vi "APC_9049_FPGA_main.vi"() -> ()   [LabVIEW 2020]
uses:
  <vilib>/Platform/TimedLoop/XDataNode/timing_clust.ctl
  <vilib>/Platform/TimedLoop/XDataNode/nitl_modes.ctl
  <vilib>/Platform/TimedLoop/XDataNode/wakeup.ctl
  <vilib>/rvi/eio/common/nirviEmuTemplateMethod_errors.vi
  <vilib>/rvi/Emulation/niFpgaGetClockAttributes.vi
  <vilib>/rvi/Emulation/niFpgaSctlEmulationGetInTimedLoop.vi
  <vilib>/rvi/Emulation/niFpgaEmulationReportErrorSimple.vi
  <vilib>/rvi/Emulation/niFpgaCriticalErrorInLSC.vi
  <vilib>/Powertrain Controls/Device Drivers/Engine Position Tracking/RevC/Encoder/FPGA/ept_enc_vte2_revc.vi
  <vilib>/eio/EIOMethodNode/EIOMethodNode.xnode
  <vilib>/eio/EIONode/EIONode.xnode
  <vilib>/Platform/TimedLoop/XDataNode/XDataNode.xnode
  <vilib>/Platform/TimedLoop/XDataNode/XDNodeRunTimeDep.lvlib
panel:
  out "Finished Late? [i-1]":bool
  out "CrankCount":u16
  out "NumberOfActiveIGN_DI":u8
  in  "manual toggle mode?":bool
  in  "Time out limit":u32=6000000
  in  "manual?":bool
  in  "PFI0 manual OUT":bool
  in  "broadcast inj+ign?":bool
  out "PFI0 DO":bool
  in  "Ticks per toggle":u32[](array[numeric])=[13000, 12000, 11000, 10000, 9000, 8000, 7000, 6000, 5000, 4000, 3000, 2000, 1000]
  in  "Toggle mode":u8
  in  "toggle TDC":bool
  in  "1/2 Z pulse":bool
  in  "Mod3/DIO7":bool
  in  "Mod3/DIO6":bool
  in  "Mod3/DIO5":bool
  in  "Mod3/DIO4":bool
  in  "Mod4/DIO7":bool
  in  "Mod4/DIO6":bool
  in  "DI 4":T1
  in  "DI 5":T1
  in  "DI 6":T1
  out "DI_Data_Mod6":T2 caption="DIData"
  in  "DI 1":T1
  in  "DI 2":T1
  in  "DI 3":T1
  in  "Spark 6":T3
  in  "Spark 5":T3
  in  "Spark 4":T3
  in  "Spark 3":T3
  in  "Spark 2":T3
  out "Cam_sim":bool
  out "EncZ_w_offset":bool
  in  "TRIG1_offset_ticks":u16=2
  in  "Cam_tooth_w_ticks":u16=8
  in  "filt_crank A_ticks":u16=2
  in  "Must Use Cam & Z":bool
  out "CamZ filt":bool
  in  "filt_cam_ticks":u16
  out "Cam":bool
  out "EncZ":bool=TRUE
  out "EncB":bool=TRUE
  out "EncA":bool
  in  "filt_crank Z_ticks":u16
  out "dT HB (ms)":u32=500
  out "dT inj (ticks)":u32=1
  out "FPGA Heartbeat":bool=TRUE
  out "Chassis Temp Raw (x4 C)":i16=140
  out "SparkOut":bool
  in  "Spark 1":T3
  in  "DI_IPhaseInterface":T4(array[cluster]) caption="IPhaseInterface"
  in  "DI_Control":T5={"ModuleEnable"=FALSE, "WatchdogIn"=TRUE, "OneShotSelect"=enum."DISABLED", "OneShotTime"=40000, "OneShot"=FALSE, "Control"=0, "Control2"=128, "HostMode"=0, "HostCommand"=0, "HVTarget"=124, "BackBoostTime"=10, "Fault_ClrSig"=FALSE} caption="DIControl"
  out "DI_Data_Mod5":T2 caption="DIData"
  out "NI9401 Ready":bool=TRUE
  out "EPTOutSig":cluster{"CrankSigOut":bool, "CamSigOut":bool}
  out "EPTData":T6={"CrankSigOS"=FALSE, "CrankStalled"=FALSE, "SyncStopped"=FALSE, "MissedCrankFlag"=FALSE, "MissedCamFlag"=FALSE, "Period"=588, "PeriodAccum"=3882066, "CrankCount"=5844, "CurrentPosition"=23376, "MAX_CAT"=57600}
  in  "EPTControl":T7={"NumberOfCrankTeeth"=7200, "Stroke (FALSE=2, TRUE=4)"=TRUE, "CrankStallPeriod"=5000000, "CrankCountStart"=7200, "PeriodAccumCount"=7200, "SyncEnable"=TRUE, "SimEnable"=FALSE, "MissedCrankFlagClr"=TRUE, "MissedCamFlagClr"=TRUE, "SimPeriod"=500, "WatchdogIn"=TRUE}
  # "This is low level FPGA interface only! - DO NOT USE DIRECTLY - Use RT module to configure"
  # "DI Control"
  # "ENCODER SIGNAL"
  # "DI Driver Settings"
  # "monarch APC v0.1"
  # "cRIO 9049 FPGA"
  # "General Monitoring & Control"
  # "USER LED1 is also \nbroadcasting the \nhearbeat at 1Hz"
  # "Additional DO"
  # "Ignition Control"
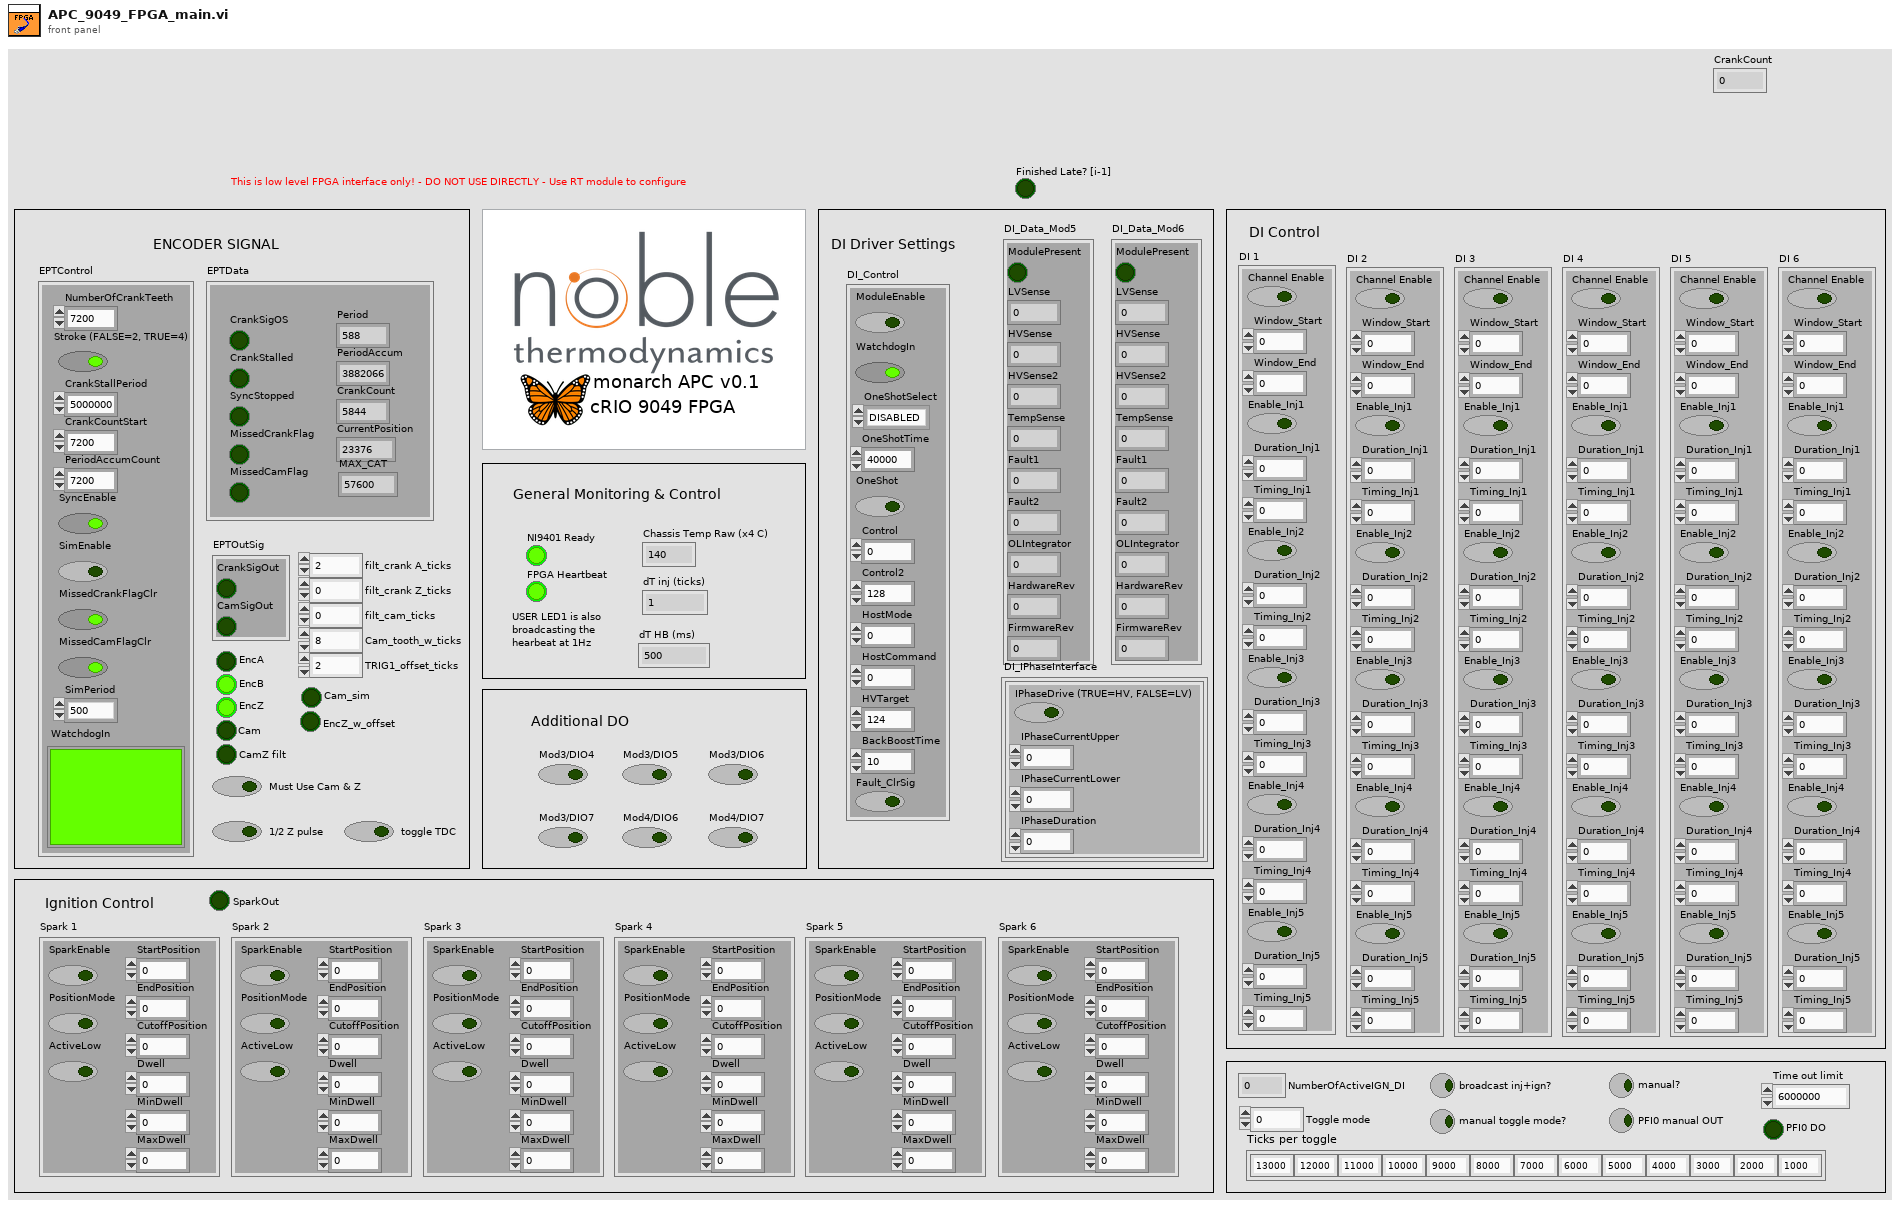
[diagram p1: front panel]
types:
  T1 = cluster{"Channel Enable":bool, "Window_Start":u16, "Window_End":u16, "Enable_Inj1":bool, "Duration_Inj1":u32, "Timing_Inj1":u16, "Enable_Inj2":bool, "Duration_Inj2":u32, "Timing_Inj2":u16, "Enable_Inj3":bool, "Duration_Inj3":u32, "Timing_Inj3":u16, "Enable_Inj4":bool, "Duration_Inj4":u32, "Timing_Inj4":u16, "Enable_Inj5":bool, "Duration_Inj5":u32, "Timing_Inj5":u16}
  T2 = cluster{"ModulePresent":bool, "LVSense":u8, "HVSense":u8, "HVSense2":u8, "TempSense":i8, "Fault1":u8, "Fault2":u8, "OLIntegrator":u32, "HardwareRev":u8, "FirmwareRev":u8}
  T3 = cluster{"SparkEnable":bool, "PositionMode":bool, "ActiveLow":bool, "StartPosition":u16, "EndPosition":u16, "CutoffPosition":u16, "Dwell":u32, "MinDwell":u32, "MaxDwell":u32}
  T4 = cluster{"IPhaseDrive (TRUE=HV, FALSE=LV)":bool, "IPhaseCurrentUpper":u16, "IPhaseCurrentLower":u16, "IPhaseDuration":u16}[]
  T5 = cluster{"ModuleEnable":bool, "WatchdogIn":bool, "OneShotSelect":enum8{"DISABLED", "CHAN 1", "CHAN 2", "CHAN 3"}, "OneShotTime":u32, "OneShot":bool, "Control":u8, "Control2":u8, "HostMode":u8, "HostCommand":u32, "HVTarget":u8, "BackBoostTime":u8, "Fault_ClrSig":bool}
  T6 = cluster{"CrankSigOS":bool, "CrankStalled":bool, "SyncStopped":bool, "MissedCrankFlag":bool, "MissedCamFlag":bool, "Period":u32, "PeriodAccum":u32, "CrankCount":u16, "CurrentPosition":u16, "MAX_CAT":u16}
  T7 = cluster{"NumberOfCrankTeeth":u16, "Stroke (FALSE=2, TRUE=4)":bool, "CrankStallPeriod":u32, "CrankCountStart":u16, "PeriodAccumCount":u16, "SyncEnable":bool, "SimEnable":bool, "MissedCrankFlagClr":bool, "MissedCamFlagClr":bool, "SimPeriod":u32, "WatchdogIn":bool}
  T8 = typedef "XDNodeRunTimeDep.lvlib/timing_clust.ctl" = cluster{"Expected End [f-1]":u64, "Actual End [f-1]":u64, "Finished Late? [f-1]":bool, "Expected End [i-1]":u64, "Actual End [i-1]":u64, "Finished Late? [i-1]":bool, "Expected Start [i]":u64, "Actual Start [i]":u64, "Expected Start [f]":u64, "Actual Start [f]":u64, "Source Name":string, "Structure Name":string, "Period":i64, "Deadline":i64, "Offset":i64, "Start":i64, "Priority":i32, "Timeout":i32, "Mode":T9, "Wakeup Reason":T10, "Error":errorcluster, "Source Type":string, "Secondary Source Type":string, "Global End Time":u64, "Global Start Time":u64, "Frame Duration":u64, "Iteration Duration":u64, "Assigned CPU":i32, "I/O Scan Engine Mode":u32}
  T9 = typedef "XDNodeRunTimeDep.lvlib/nitl_modes.ctl" = enum32{"No Change", "Process missed periods, maintain original phase", "Discard missed periods, maintain original phase", "Process missed periods, ignore original phase", "Discard missed periods, ignore original phase"}
  T10 = typedef "XDNodeRunTimeDep.lvlib/wakeup.ctl" = enum32{"Normal", "Aborted", "Asynchronous wakeup", "Timing source error", "Timed loop error", "Timeout"}
  T11 = cluster{"FSSup0":bool, "FSSup1":bool, "FSSup2":bool, "FSSup3":u16, "FSSup4":u32, "FSSup5":u16}
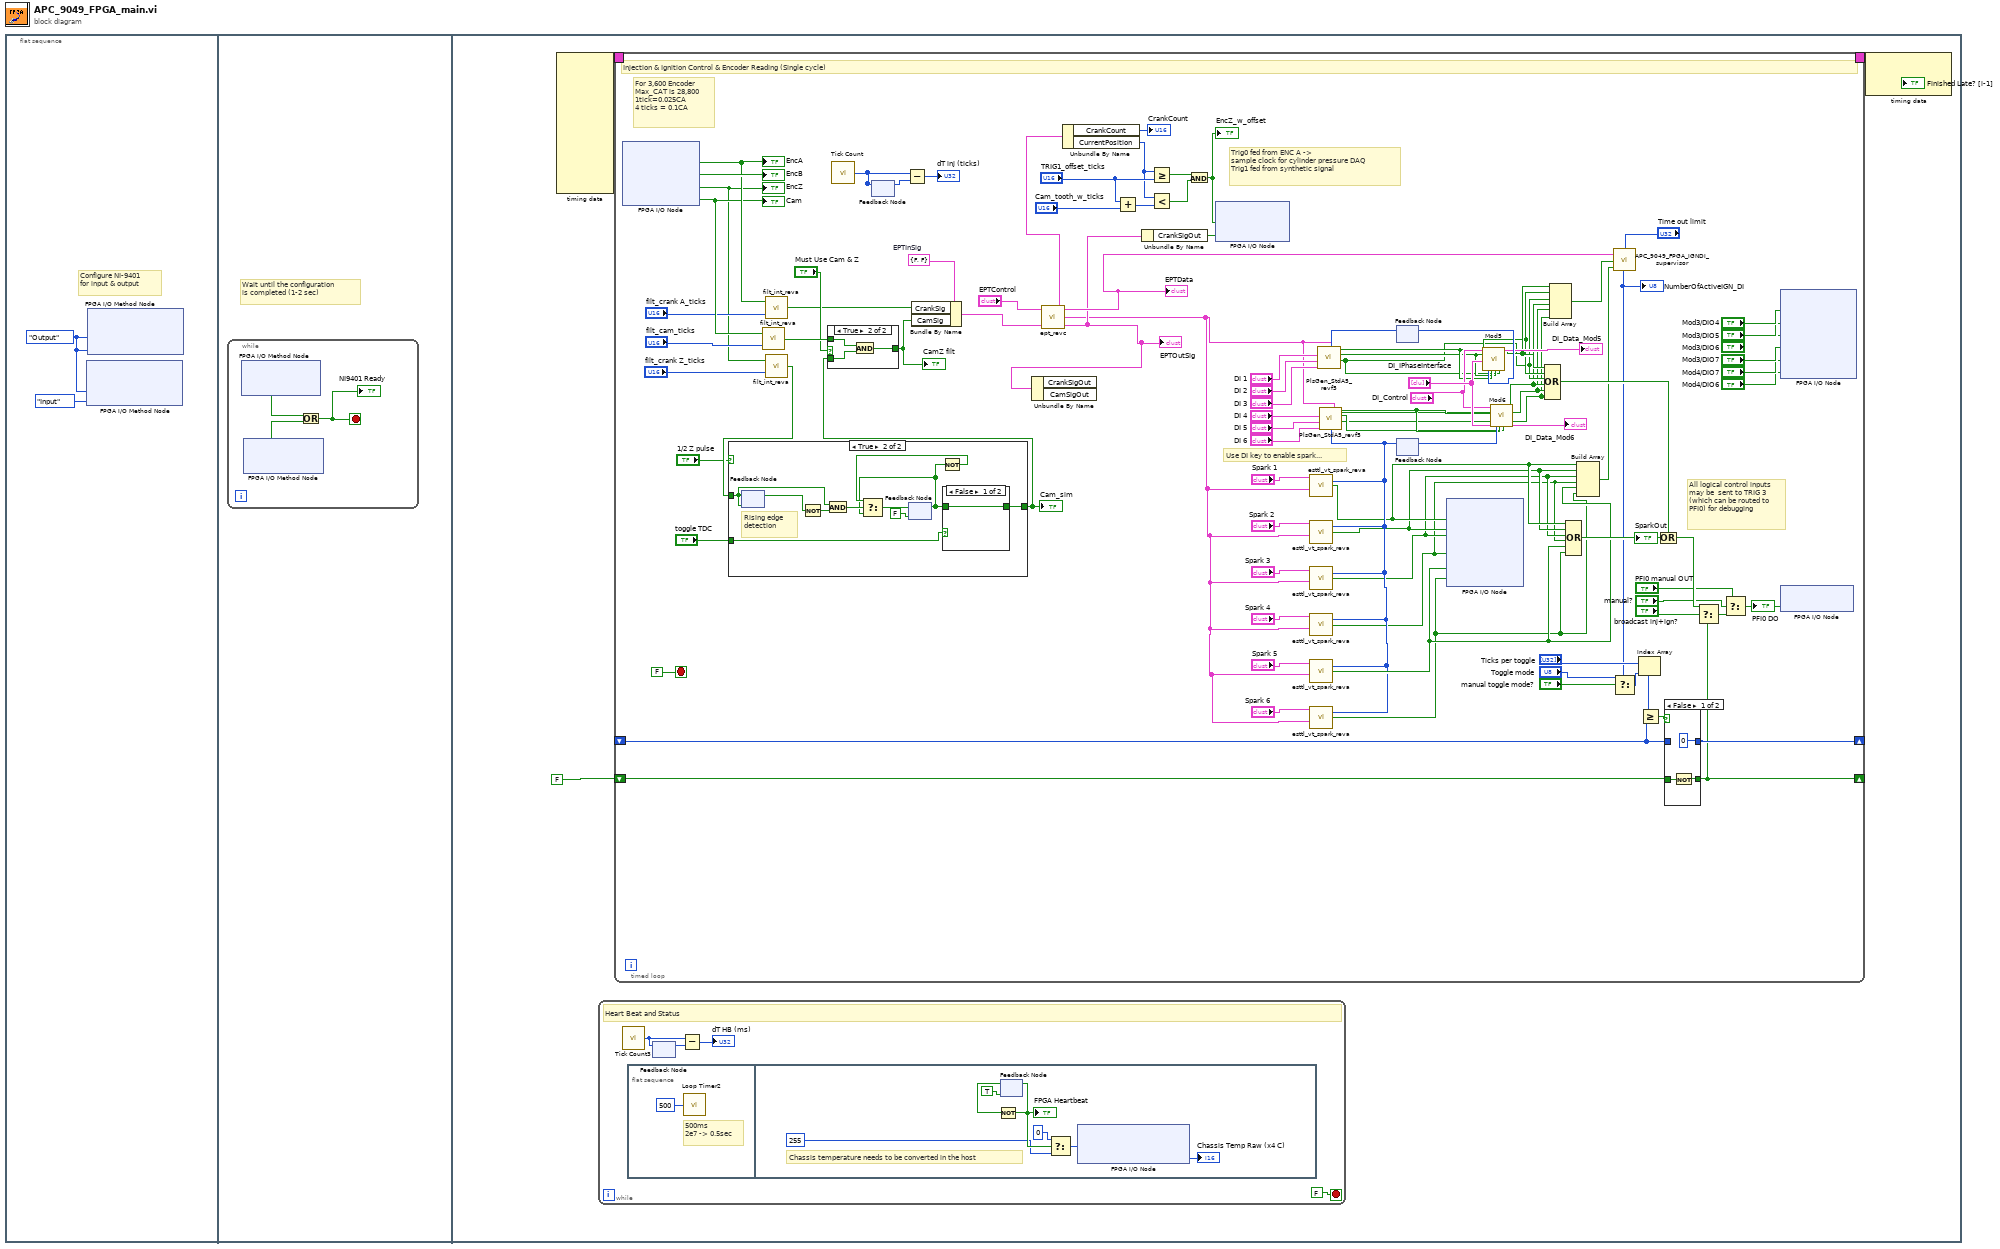
[diagram p0: block diagram]
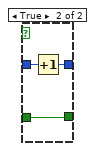
[diagram p2: hidden frame]
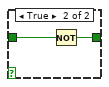
[diagram p4: hidden frame]
diagram:
  n1 = flat-sequence {
    frame #0 {
      w1 = enum8{"No Change", "Input", "Output"}."Output" ("DIO 7:4")
      # "Configure NI-9401 \nfor input & output"
      n2 = xnode "FPGA I/O Method Node"("DIO 7:4"=w1, "DIO 3:0"=enum8{"No Change", "Input", "Output"}."Input" ("DIO 7:4")) -> ()  [unwired: 1 in, 1 out]
      n3 = xnode "FPGA I/O Method Node"("DIO 7:4"=w1, "DIO 3:0"=w1) -> ()  [unwired: 1 in, 1 out]
    }
    frame #1 {
      # "Wait until the configuration \nis completed (1-2 sec)"
      n4 = while {
        stop <- w3 stop-if-true
        n5 = xnode "FPGA I/O Method Node"() -> ("Ready"=w5:bool)  [unwired: 1 in, 1 out]
        n6 = xnode "FPGA I/O Method Node"() -> ("Ready"=w4:bool)  [unwired: 1 in, 1 out]
        n7 = Or(x=w5, y=w4) -> (x .or. y?=w3:bool)
        "NI9401 Ready" <- w3
      }
    }
    frame #2 {
      n8 = node-c288() -> (w9:T8)  [unwired: 10 in]
      n9 = while {
        stop <- FALSE stop-if-true
        # "Heart Beat and Status"
        n10 = call "Tick Count3"() -> ("Tick Count(mSec)"=w12:u16)
        n11 = flat-sequence {
          frame #0 {
            # "500ms\n2e7 -> 0.5sec"
            n12 = call "Loop Timer2"("Count(mSec)"=u32 500) -> ()  [unwired: 1 out]
          }
          frame #1 {
            # "Chassis temperature needs to be converted in the host"
            n13 = feedback #1(TRUE ("USER FPGA LED")) -> (w19:bool)
            n14 = Not(x=w19) -> (.not. x?=w18:bool)
            "FPGA Heartbeat" <- w18
            n15 = feedback-in #1(w18) -> ()
            n16 = Select(t=u8 0, s=w18, f=u8 255) -> (s? t:f=w17:u8)
            n17 = xnode "FPGA I/O Node"("USER FPGA LED"=w17) -> ("Chassis Temperature"=→"Chassis Temp Raw (x4 C)":i16)  [unwired: 2 in, 2 out]
          }
        }
        n18 = feedback #2() -> (w13:u16)  [unwired: 1 in]
        n19 = feedback-in #2(w12) -> ()
        n20 = Subtract(x=w12, y=w13) -> (x-y=→"dT HB (ms)":u16)
      }
      n21 = timed-loop {
        timing-out: [_] -> w8
        timing: w9 -> [_]
        shift-right: [w73] -> _
        shift-left: _ -> [w72]
        shift-right: [w45] -> _
        shift-left: FALSE ("PFI0 mode signal") -> [w71]
        stop <- FALSE stop-if-true
        w109 = cluster{"CrankSig":bool, "CamSig":bool} {"CrankSig"=FALSE, "CamSig"=FALSE}  # EPTInSig
        # "All logical control inputs may be  sent to TRIG 3 (which can be routed to PFI0) for debugging"
        # "For 3,600 Encoder\nMax_CAT is 28,800\n1tick=0.025CA\n4 ticks = 0.1CA"
        # "Trig0 fed from ENC A -> \nsample clock for cylinder pressure DAQ\nTrig1 fed from synthetic signal"
        # "Use DI key to enable spark..."
        # "Injection & Ignition Control & Encoder Reading (Single cycle)"
        n22 = xnode "FPGA I/O Node"() -> ("Mod3/DIO0"=w107:bool, "Mod3/DIO1"=→"EncB":bool, "Mod3/DIO2"=w92:bool, "Mod3/DIO3"=w106:bool)  [unwired: 4 in, 4 out]
        "EncA" <- w107
        "EncZ" <- w92
        "Cam" <- w106
        n23 = call <vilib>:"filt_int_reva.vi"("FiltValue"="filt_cam_ticks", "InpSig"=w106) -> ("OutSig"=w103:bool)
        n24 = call <vilib>:"filt_int_reva.vi"("FiltValue"="filt_crank A_ticks", "InpSig"=w107) -> ("OutSig"=w38:bool)
        n25 = call <vilib>:"filt_int_reva.vi"("FiltValue"="filt_crank Z_ticks", "InpSig"=w92) -> ("OutSig"=w91:bool)
        n26 = case shown="True" "1/2 Z pulse" {
          tunnel: w91 -> [w122 w127]
          tunnel: [w122 w123] -> w40
          tunnel: "toggle TDC" -> [_ w125]
          frame False {
          }
          frame True {
            # "Rising edge \ndetection"
            n27 = feedback #3(w127) -> (w132:bool)
            n28 = feedback-in #3(w127) -> ()
            n29 = Not(x=w132) -> (.not. x?=w131:bool)
            n30 = And(x=w127, y=w131) -> (x .and. y?=w126:bool)
            n31 = feedback #4(FALSE) -> (w124:bool)
            n32 = Not(x=w124) -> (.not. x?=w130:bool)
            n33 = Select(t=w130, s=w126, f=w124) -> (s? t:f=w129:bool)
            n34 = feedback-in #4(w129) -> ()
            n35 = case shown="False" w125 {
              tunnel: w124 -> [w133 w135]
              tunnel: [w133 w134] -> w123
              frame False {
              }
              frame True {
                n36 = Not(x=w135) -> (.not. x?=w134:bool)
              }
            }
          }
        }
        "Cam_sim" <- w40
        n37 = case shown="True" "Must Use Cam & Z" {
          tunnel: w103 -> [_ w139]
          tunnel: w40 -> [w136 w138]
          tunnel: [w136 w137] -> w39
          frame False {
          }
          frame True {
            n38 = And(x=w139, y=w138) -> (x .and. y?=w137:bool)
          }
        }
        "CamZ filt" <- w39
        n39 = call "Tick Count"() -> ("Tick Count(Ticks)"=w112:u32)
        n40 = feedback-in #5(w112) -> ()
        n41 = feedback #5(w112) -> (w113:u32)
        n42 = Subtract(x=w112, y=w113) -> (x-y=→"dT inj (ticks)":u32)
        n43 = Bundle By Name(cluster=w109, "CrankSig"=w38, "CamSig"=w39) -> (w108:cluster{"CrankSig":bool, "CamSig":bool})
        n44 = call-poly <vilib>:"ept_revc.vi"("EPTControl"="EPTControl", "EPTInSig"=w108) -> ("EPTData"=w47:T6, "FuelSparkSupervisor"=w22:T11, "EPTOutSig"=w37:cluster{"CrankSigOut":bool, "CamSigOut":bool})  [unwired: 3 in]
        "EPTData" <- w47
        "EPTOutSig" <- w37
        n45 = Unbundle By Name(w37) -> ()  [unwired: 2 out]
        n46 = Unbundle By Name(w47) -> ("CrankCount"=→"CrankCount":u16, "CurrentPosition"=w97:u16)
        n47 = Add(x="TRIG1_offset_ticks", y="Cam_tooth_w_ticks") -> (x+y=w96:u16)
        n48 = Unbundle By Name(w37) -> ("CrankSigOut"=w35:bool)
        n49 = Greater Or Equal?(x=w97, y="TRIG1_offset_ticks") -> (x >= y?=w95:bool)
        n50 = Less?(x=w97, y=w96) -> (x < y?=w94:bool)
        n51 = And(x=w95, y=w94) -> (x .and. y?=w93:bool)
        "EncZ_w_offset" <- w93
        n52 = xnode "FPGA I/O Node"("cRIO_Trig1"=w93, "cRIO_Trig0"=w35) -> ()  [unwired: 2 in, 2 out]
        n53 = feedback #6() -> (w57:u16)  [unwired: 1 in]
        n54 = call <vilib>:"PlsGen_StdA5_revf5.vi"("PlsGen_Config_Channel3"="DI 3", "PlsGen_Config_Channel2"="DI 2", "PlsGen_Config_Channel1"="DI 1", "key"=w57, "FuelSparkSupervisor"=w22) -> ("CmdOut3"=w54:bool, "CmdOut2"=w55:bool, "CmdOut1"=w56:bool)  [unwired: 2 in]
        n55 = feedback #7() -> (w34:u16)  [unwired: 1 in]
        n56 = call <vilib>:"esttl_vt_spark_reva.vi"("SparkControl"="Spark 1", "Key"=w34, "FuelSparkSupervisor"=w22) -> ("SparkOut"=w27:bool)  [unwired: 5 in]
        n57 = call <vilib>:"esttl_vt_spark_reva.vi"("SparkControl"="Spark 2", "Key"=w34, "FuelSparkSupervisor"=w22) -> ("SparkOut"=w26:bool)  [unwired: 5 in]
        n58 = call <vilib>:"esttl_vt_spark_reva.vi"("SparkControl"="Spark 3", "Key"=w34, "FuelSparkSupervisor"=w22) -> ("SparkOut"=w25:bool)  [unwired: 5 in]
        n59 = call <vilib>:"esttl_vt_spark_reva.vi"("SparkControl"="Spark 4", "Key"=w34, "FuelSparkSupervisor"=w22) -> ("SparkOut"=w24:bool)  [unwired: 5 in]
        n60 = call <vilib>:"esttl_vt_spark_reva.vi"("SparkControl"="Spark 5", "Key"=w34, "FuelSparkSupervisor"=w22) -> ("SparkOut"=w50:bool)  [unwired: 5 in]
        n61 = call <vilib>:"esttl_vt_spark_reva.vi"("SparkControl"="Spark 6", "Key"=w34, "FuelSparkSupervisor"=w22) -> ("SparkOut"=w23:bool)  [unwired: 5 in]
        n62 = call <vilib>:"PlsGen_StdA5_revf5.vi"("PlsGen_Config_Channel3"="DI 6", "PlsGen_Config_Channel2"="DI 5", "PlsGen_Config_Channel1"="DI 4", "key"=w34, "FuelSparkSupervisor"=w22) -> ("CmdOut3"=w51:bool, "CmdOut2"=w52:bool, "CmdOut1"=w53:bool)  [unwired: 2 in]
        n63 = xnode "FPGA I/O Node"("Mod4/DIO0"=w27, "Mod4/DIO1"=w26, "Mod4/DIO2"=w25, "Mod4/DIO3"=w24, "Mod4/DIO4"=w50, "Mod4/DIO5"=w23) -> ()  [unwired: 6 in, 6 out]
        n64 = call "Mod5"("Mod5_Control"="DI_Control", "Mod5_IPhaseInterface"="DI_IPhaseInterface", "DI1Cmd"=w56, "DI2Cmd"=w55, "DI3Cmd"=w54) -> ("Key Out"=w114:u16, "Mod5_Data"=→"DI_Data_Mod5":T2)  [unwired: 12 in, 1 out]
        n65 = feedback-in #6(w114) -> ()
        n66 = call "Mod6"("Mod6_Control"="DI_Control", "Mod6_IPhaseInterface"="DI_IPhaseInterface", "DI1Cmd"=w53, "DI2Cmd"=w52, "DI3Cmd"=w51) -> ("Key Out"=w80:u16, "Mod6_Data"=→"DI_Data_Mod6":T2)  [unwired: 12 in, 1 out]
        n67 = feedback-in #7(w80) -> ()
        n68 = Compound Arithmetic op=OR(w56, w55, w54, w53, w52, w51) -> (w77:bool)
        n69 = Build Array(w56, w55, w54, w53, w52, w51) -> (w49:bool[])
        n70 = Compound Arithmetic op=OR(w27, w26, w25, w24, w50, w23) -> (w64:bool)
        "SparkOut" <- w64
        n71 = Build Array(w27, w26, w25, w24, w50, w23) -> (w48:bool[])
        n72 = call "APC_9049_FPGA_IGNDI_supervisor.vi"("Time out limit"="Time out limit", "EPTData"=w47, "SIarray"=w48, "DIarray"=w49) -> ("NumberOfActiveIGN_DI"=w44:u8)
        "NumberOfActiveIGN_DI" <- w44
        n73 = Select(t="Toggle mode", s="manual toggle mode?", f=w44) -> (s? t:f=w41:u8)
        n74 = Index Array(array="Ticks per toggle", index=w41) -> (element=w75:u32)
        n75 = Greater Or Equal?(x=w75, y=w72) -> (x >= y?=w74:bool)
        n76 = Or(x=w77, y=w64) -> (x .or. y?=w70:bool)
        n77 = case shown="False" w74 {
          tunnel: [u32 0 ("Ticks per toggle") w121] -> w73
          tunnel: w72 -> [_ w120]
          tunnel: w71 -> [w117 w119]
          tunnel: [w116 w119] -> w45
          frame False {
            n78 = Not(x=w117) -> (.not. x?=w116:bool)
          }
          frame True {
            n79 = Increment(x=w120) -> (x+1=w121:u32)
          }
        }
        n80 = Select(t=w70, s="broadcast inj+ign?", f=w45) -> (s? t:f=w68:bool)
        n81 = Select(t="PFI0 manual OUT", s="manual?", f=w68) -> (s? t:f=w65:bool)
        "PFI0 DO" <- w65
        n82 = xnode "FPGA I/O Node"("Mod3/DIO4"="Mod3/DIO4", "Mod3/DIO5"="Mod3/DIO5", "Mod3/DIO6"="Mod3/DIO6", "Mod3/DIO7"="Mod3/DIO7", "Mod4/DIO6"="Mod4/DIO7", "Mod4/DIO7"="Mod4/DIO6") -> ()  [unwired: 6 in, 6 out]
        n83 = xnode "FPGA I/O Node"("cRIO_Trig3"=w65) -> ()  [unwired: 1 in, 1 out]
      }
      n84 = node-c288(w8) -> (→"Finished Late? [i-1]":bool)  [unwired: 1 out]
    }
  }
